vi "Input Box GUI.vi"(8 "error in":errorcluster, 10 "Default Input":refnum<class "UTF-8 String.lvclass">, 11 "Message":refnum<class "UTF-8 String.lvclass">) -> (0 "error out":errorcluster, 2 "Input":refnum<class "UTF-8 String.lvclass">, 3 "Cancelled":bool)   [LabVIEW 2020, in "G-Unicode.lvlib"]
doc: "Displays a dialog box where the user can input a string."
uses:
  G-Unicode.lvlib
  Types/UTF-8 String/UTF-8 String.lvclass
  a6561194-ee96-4257-99bb-cbad27b49c54.vi
  8c6cc9e0-8059-4770-9006-a9bd928332ac.vi
  Types/Encoded UTF-8 String.ctl
  Dialog & User Interface/Polymorphic VIs/Read Control Text/Read String Value (UTF-8 String).vi
  Dialog & User Interface/Polymorphic VIs/Write Control Text/Write String Value (UTF-8 String).vi
panel:
  in  "User Input":string caption="Text input:"
  in  "Cancel":bool
  in  "OK":bool
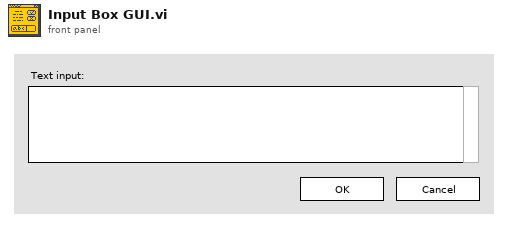
[diagram p1: front panel]
types:
  T1 = typedef "G-Unicode.lvlib/Encoded UTF-8 String.ctl" = string
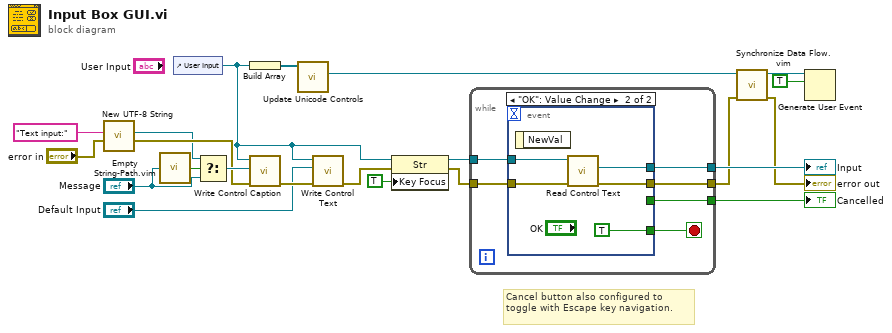
[diagram p0: block diagram]
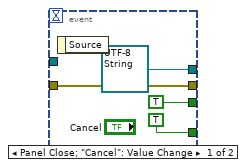
[diagram p2: hidden frame]
diagram:
  # "Cancel button also configured to toggle with Escape key navigation."
  n1 = call "New UTF-8 String.vi"("error in"="error in", "String"=T1 "Text input:" ("LabVIEW String")) -> ("error out"=w3:errorcluster, "UTF-8 String"=w2:refnum<class "UTF-8 String.lvclass">)  [unwired: 8 in]
  n2 = call "Empty String-Path.vim"("String/Path"="Message") -> ("Empty?"=w6:bool)
  n3 = control-ref of="User Input"() -> (w1:refnum<vi>)
  n4 = Select(t=w2, s=w6, f="Message") -> (s? t:f=w8:refnum<class "UTF-8 String.lvclass">)
  n5 = Build Array(w1) -> (w22:refnum<vi>[])
  n6 = call "Write Control Caption.vi"("error in"=w3, "Text"=w8, "Control Ref"=w1) -> ("error out"=w21:errorcluster)  [unwired: 8 in]
  n7 = call "Update Unicode Controls.vi"("String Refs"=w22) -> ("Stop Event"=w18:refnum<user-event>)  [unwired: 8 in, 2 out]
  n8 = call-poly "Write Control Text.vi"("error in"=w21, "Value"="Default Input", "Control Ref"=w1) -> ("error out"=w11:errorcluster)  [unwired: 8 in]
  n9 = property class="Str"(reference=w1, error in=w11, "Key Focus"=TRUE) -> (reference out=w13:refnum<vi>, error out=w10:errorcluster)
  n10 = while {
    tunnel: [w28] -> w20
    tunnel: [w27] -> w19
    tunnel: w13 -> [w26]
    tunnel: w10 -> [w25]
    tunnel: [w24] -> w16
    stop <- w23 stop-if-true
    n11 = event shown="[1] \"OK\": Value Change" {
      selector: _ -> [_ _]
      dyn-events: _ -> [_ _]
      timeout: _ -> [_ _]
      tunnel: [refnum<class "UTF-8 String.lvclass"> refnum ("Input") w37] -> w28
      tunnel: [TRUE _] -> w27
      tunnel: w26 -> [_ w34]
      tunnel: w25 -> [w29 w33]
      tunnel: [w29 w36] -> w24
      tunnel: [TRUE TRUE] -> w23
      event Panel Close; "Cancel": Value Change {
        n12 = event-data() -> ()  [unwired: 1 in, 1 out]
      }
      event "OK": Value Change {
        n13 = event-data() -> ()  [unwired: 1 in, 1 out]
        n14 = call-poly "Read Control Text.vi"("error in"=w33, "Control Ref"=w34) -> ("error out"=w36:errorcluster, "UTF-8 String"=w37:refnum<class "UTF-8 String.lvclass">)  [unwired: 8 in]
      }
    }
  }
  "Input" <- w20
  "Cancelled" <- w19
  n15 = call "Synchronize Data Flow.vim"("input 4"=w16, "input 1"=w18) -> ("output 4"=→"error out":errorcluster, "output 1"=w17:refnum<user-event>)  [unwired: 2 in, 2 out]
  n16 = Generate User Event(user event=w17, event data cluster=TRUE ("event data")) -> ()  [unwired: 2 in, 2 out]
